vi "PWM_Motor_IR.vi"(0 "Sensor schräg rechts":dbl, 5 "Sensor schräg  links":dbl, 7 "Sensor geradeaus rechts":dbl, 9 "Sensor geradeaus links":dbl, 11 "Motor multiplikator":dbl) -> (3 "Folgen?":bool, 4 "PWM Motor":dbl=0.3)   [LabVIEW 2016]
doc: "Geschwindigkeitsregelung anhand IR Sensor vorne\n05.04.17_Tloe"
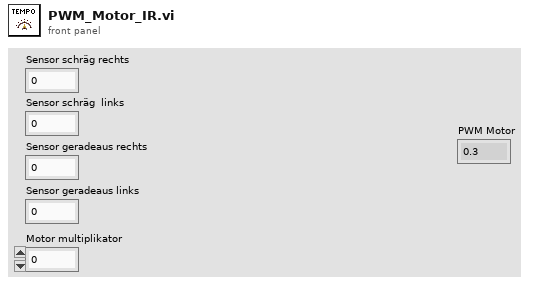
[diagram p1: front panel]
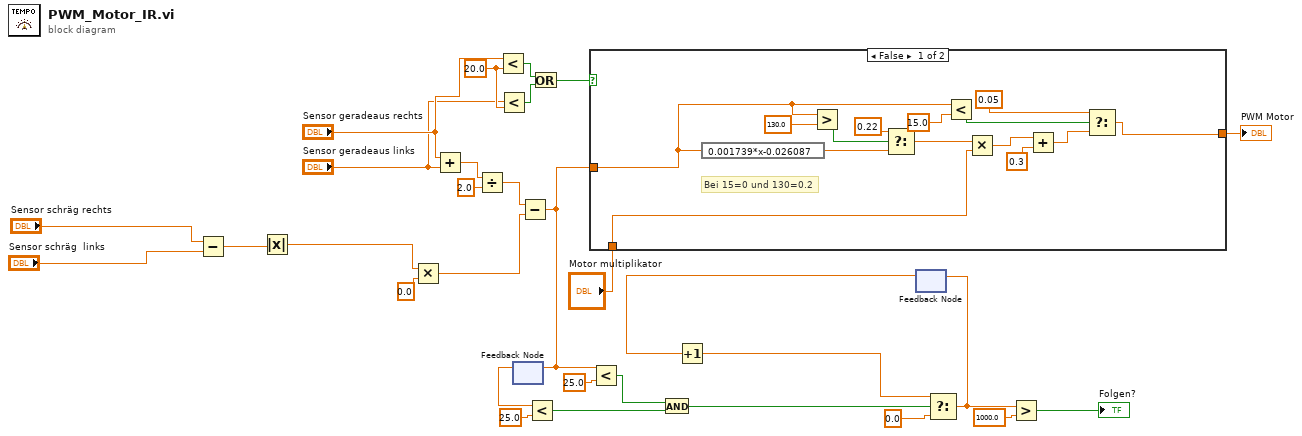
[diagram p0: block diagram]
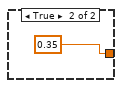
[diagram p2: hidden frame]
diagram:
  w8 = 20.0 ("y")
  n1 = Subtract(x="Sensor schräg rechts", y="Sensor schräg  links") -> (x-y=w11:dbl)
  n2 = Absolute Value(x=w11) -> (abs(x)=w10:dbl)
  n3 = Multiply(x=w10, y=0.0) -> (x*y=w12:dbl)
  n4 = Add(x="Sensor geradeaus rechts", y="Sensor geradeaus links") -> (x+y=w16:dbl)
  n5 = Divide(x=w16, y=2.0) -> (x/y=w14:dbl)
  n6 = Less?(x="Sensor geradeaus rechts", y=w8) -> (x < y?=w6:bool)
  n7 = Less?(x="Sensor geradeaus links", y=w8) -> (x < y?=w5:bool)
  n8 = feedback #1() -> (w30:dbl)  [unwired: 1 in]
  n9 = Subtract(x=w14, y=w12) -> (x-y=w2:dbl)
  n10 = feedback-in #1(w2) -> ()
  n11 = Less?(x=w30, y=25.0) -> (x < y?=w26:bool)
  n12 = Or(x=w6, y=w5) -> (x .or. y?=w3:bool)
  n13 = case shown="False" w3 {
    tunnel: w2 -> [w32 _]
    tunnel: [w33 0.35 ("t")] -> w4
    tunnel: "Motor multiplikator" -> [w31 _]
    frame False {
      # "Bei 15=0 und 130=0.2"
      n14 = expression code="0.001739*x-0.026087"(w32) -> (w38:dbl)
      n15 = Greater?(x=w32, y=130.0) -> (0:w43:bool)
      n16 = Select(t=0.22, s=w43, f=w38) -> (s? t:f=w40:dbl)
      n17 = Less?(x=w32, y=15.0) -> (x < y?=w36:bool)
      n18 = Multiply(x=w40, y=w31) -> (x*y=w41:dbl)
      n19 = Add(x=w41, y=0.3) -> (x+y=w37:dbl)
      n20 = Select(t=0.05, s=w36, f=w37) -> (s? t:f=w33:dbl)
    }
    frame True {
    }
  }
  "PWM Motor" <- w4
  n21 = Less?(x=w2, y=25.0) -> (x < y?=w27:bool)
  n22 = And(x=w27, y=w26) -> (x .and. y?=w25:bool)
  n23 = feedback #2() -> (w22:dbl)  [unwired: 1 in]
  n24 = Increment(x=w22) -> (x+1=w23:dbl)
  n25 = Select(t=w23, s=w25, f=0.0) -> (s? t:f=w21:dbl)
  n26 = feedback-in #2(w21) -> ()
  n27 = Greater?(x=w21, y=1000.0) -> (0:→"Folgen?":bool)
